vi "StreamEngine.Main.Stream.Read.vi"(8 "error in (no error)":errorcluster, 10 "SubProcesses":T2, 11 "gRPC ID":T1) -> (0 "error out":errorcluster, 2 "Success":bool, 3 "gRPC ID out":T1)   [LabVIEW 2025, in "XNET Bus Monitor Client.lvlib"]
uses:
  XNET Bus Monitor Client.lvlib
  xnet_can_bus_monitor_api_client/xnet_can_bus_monitor_api_client.lvlib
  Types/SubProcessEngine.CmdQueueData.Cmd.ctl
  Types/SubProcessEngine.CmdQueueData.ctl
  xnet_can_bus_monitor_api_client/RPC Messages/ni_xnet_can_bm_api_CommState.ctl
  xnet_can_bus_monitor_api_client/RPC Messages/ni_xnet_can_bm_api_LastCommError.ctl
  xnet_can_bus_monitor_api_client/RPC Messages/ni_xnet_can_bm_api_CanCommState.ctl
  xnet_can_bus_monitor_api_client/RPC Messages/ni_xnet_can_bm_api_Frame.ctl
  xnet_can_bus_monitor_api_client/RPC Messages/ni_xnet_can_bm_api_ErrorInfo.ctl
  xnet_can_bus_monitor_api_client/RPC Messages/ni_xnet_can_bm_api_StreamBusReply.ctl
  Types/SubProcessEngine.CmdQueueData.Publish.ctl
  <vilib>/gRPC/LabVIEW gRPC Library/Shared/grpcId.ctl
  <vilib>/gRPC/LabVIEW gRPC Library/grpc-lvsupport-release.lvlib
  Types/SubProcessEngine.QueueRefs.ctl
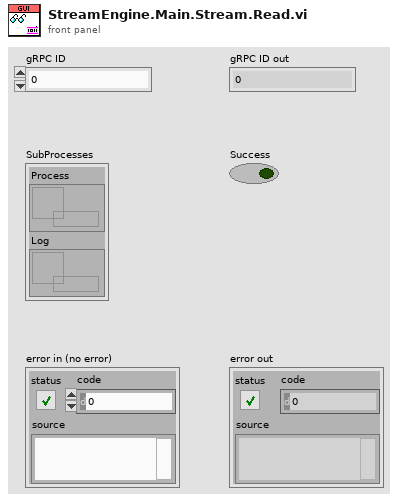
[diagram p1: front panel]
types:
  T1 = typedef "grpc-lvsupport-release.lvlib/grpcId.ctl" = u64
  T2 = typedef "XNET Bus Monitor Client.lvlib/SubProcessEngine.QueueRefs.ctl" = cluster{"Process":refnum<queue>, "Log":refnum<queue>}
  T3 = typedef "xnet_can_bus_monitor_api_client.lvlib/ni_xnet_can_bm_api_StreamBusReply.ctl" = cluster{"can_comm_state":T4, "frame":T7[], "error":T8}
  T4 = typedef "xnet_can_bus_monitor_api_client.lvlib/ni_xnet_can_bm_api_CanCommState.ctl" = cluster{"fault_code":i32, "fault":bool, "comm_state":T5, "last_comm_error":T6, "receive_error_counter":u32, "transmit_error_counter":u32, "transceiver_error":bool, "sleep":bool}
  T5 = typedef "xnet_can_bus_monitor_api_client.lvlib/ni_xnet_can_bm_api_CommState.ctl" = enum32{"Error_Active", "Error_Passive", "Bus_Off", "Init"}
  T6 = typedef "xnet_can_bus_monitor_api_client.lvlib/ni_xnet_can_bm_api_LastCommError.ctl" = enum32{"None", "Stuff", "Form", "ACK", "Bit1", "Bit0", "CRC"}
  T7 = typedef "xnet_can_bus_monitor_api_client.lvlib/ni_xnet_can_bm_api_Frame.ctl" = cluster{"timestamp":dbl, "payload":u8[], "identifier":u32, "frame_type":u32, "extended":bool, "echo":bool}
  T8 = typedef "xnet_can_bus_monitor_api_client.lvlib/ni_xnet_can_bm_api_ErrorInfo.ctl" = errorcluster
  T9 = typedef "XNET Bus Monitor Client.lvlib/SubProcessEngine.CmdQueueData.Publish.ctl" = cluster{"Response Data":T3, "Success":bool}
  T10 = typedef "XNET Bus Monitor Client.lvlib/SubProcessEngine.CmdQueueData.ctl" = cluster{"Cmd":T11, "Parameters":variant}
  T11 = typedef "XNET Bus Monitor Client.lvlib/SubProcessEngine.CmdQueueData.Cmd.ctl" = enum16{"Arm", "Publish", "Stop", "Exit"}
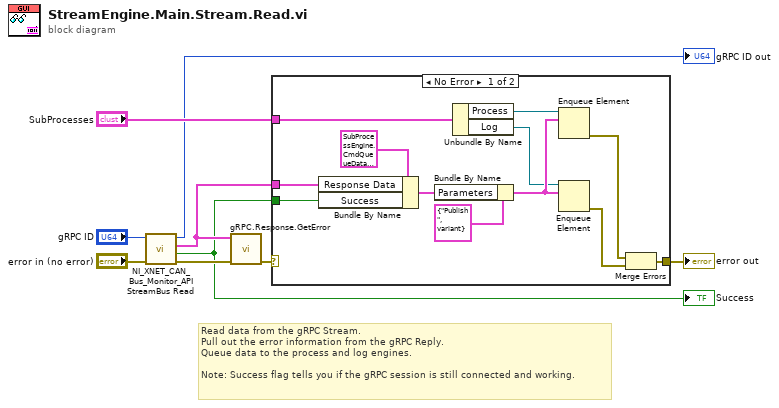
[diagram p0: block diagram]
diagram:
  # "Read data from the gRPC Stream.\nPull out the error information from the gRPC Reply.\nQueue data to the process and log engines.\n\nNote: Success flag tells you if the gRPC session is still connected and working."
  n1 = call "NI_XNET_CAN_Bus_Monitor_API StreamBus Read.vi"("error in"="error in (no error)", "Call ID in"="gRPC ID") -> ("error out"=w9:errorcluster, "Success"=w1:bool, "Response Data"=w7:T3, "Call ID"=→"gRPC ID out":T1)  [unwired: 6 in]
  "Success" <- w1
  n2 = call "gRPC.Response.GetError.vi"("error in (no error)"=w9, "Response"=w7) -> ("error out"=w3:errorcluster)  [unwired: 9 in]
  n3 = case shown="No Error" w3 {
    selector: w3 -> [_ w22]
    tunnel: [w14 w22] -> w2
    tunnel: w7 -> [w11 _]
    tunnel: "SubProcesses" -> [w19 _]
    tunnel: w1 -> [w13 _]
    frame No Error {
      n4 = Bundle By Name(cluster=T9 {"Response Data"={"can_comm_state"={"fault_code"=0, "fault"=FALSE, "comm_state"=enum."Error_Active", "last_comm_error"=enum."None", "receive_error_counter"=0, "transmit_error_counter"=0, "transceiver_error"=FALSE, "sleep"=FALSE}, "frame"=[], "error"={"status"=FALSE, "code"=0, "source"=""}}, "Success"=FALSE}, "Response Data"=w11, "Success"=w13) -> (w12:T9)
      n5 = Bundle By Name(cluster=T10 {"Cmd"=enum."Publish", "Parameters"=variant} ("element"), "Parameters"=w12) -> (w20:T10)
      n6 = Unbundle By Name(w19) -> ("Process"=w18:refnum<queue>, "Log"=w17:refnum<queue>)
      n7 = Enqueue Element(queue=w18, element=w20) -> (error out=w16:errorcluster)  [unwired: 2 in, 2 out]
      n8 = Enqueue Element(queue=w17, element=w20) -> (error out=w15:errorcluster)  [unwired: 2 in, 2 out]
      n9 = Merge Errors(w16, w15) -> (w14:errorcluster)
    }
    frame Error {
    }
  }
  "error out" <- w2
